vi "Configure Frequency Sweep.vi"(8 "error in (no error)":errorcluster, 10 "Freq Sweep Setting":T1={"Sweep Spacing (0: Linear)"=0, "Sweep Time (1.00 s)"=1.0, "Stop  Frequency (1000.0 Hz)"=1000.0, "Start Frequency (100.0 Hz)"=100.0, "Enable/Disable Freq Sweep"=FALSE} {"Start Frequency (100.0 Hz)" format="%#.6g"; "Stop  Frequency (1000.0 Hz)" format="%#.6g"; "Sweep Time (1.00 s)" format="%#.6g"; "Sweep Spacing (0: Linear)" items=["Linear", "Logarithmic"]}, 11 "Abstract in":refnum<class "Abstract.lvclass">) -> (0 "error out":errorcluster, 3 "Abstract out":refnum<class "Abstract.lvclass">)   [LabVIEW 2023, in "Func Generator.lvlib" / "Abstract.lvclass"]
uses:
  Abstract.lvclass
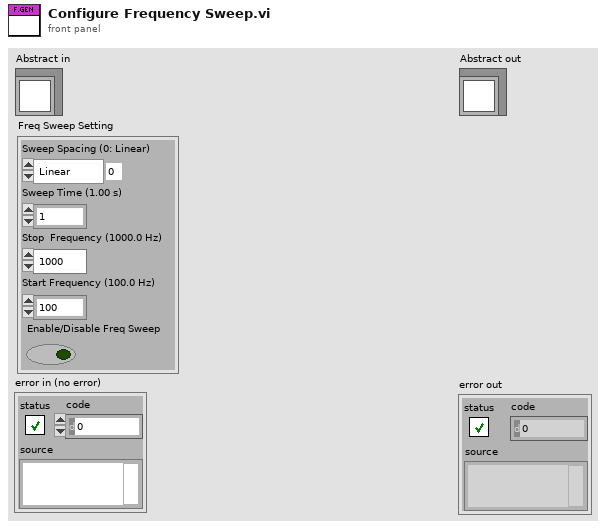
[diagram p1: front panel]
types:
  T1 = cluster{"Sweep Spacing (0: Linear)":u16, "Sweep Time (1.00 s)":dbl, "Stop  Frequency (1000.0 Hz)":dbl, "Start Frequency (100.0 Hz)":dbl, "Enable/Disable Freq Sweep":bool}
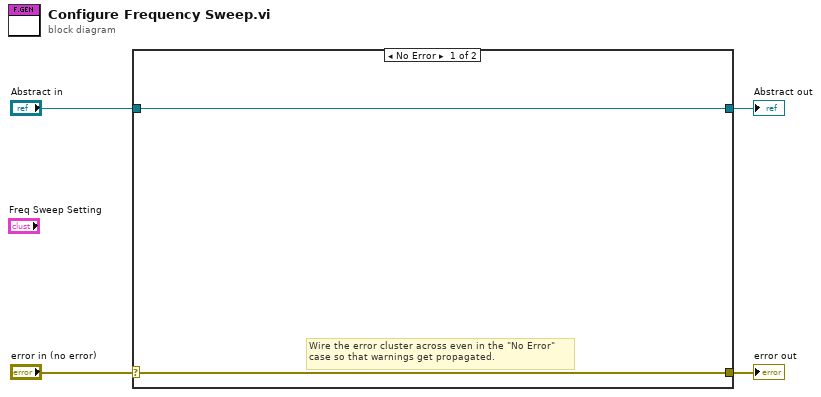
[diagram p0: block diagram]
diagram:
  n1 = case shown="No Error" "error in (no error)" {
    selector: "error in (no error)" -> [w5 w8]
    tunnel: [w5 w8] -> w3
    tunnel: [w6 w7] -> w1
    tunnel: "Abstract in" -> [w6 w7]
    frame No Error {
      # "Wire the error cluster across even in the \"No Error\"\ncase so that warnings get propagated."
    }
    frame Error {
    }
  }
  "error out" <- w3
  "Abstract out" <- w1
